vi "GageVolScale.vi"(2 "Voltage Scale":u16(ring)=4) -> (1 "Scaling Factor":dbl format="%.2f")   [LabVIEW 2022 SP3]
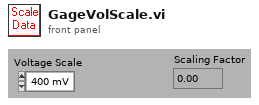
[diagram p1: front panel]
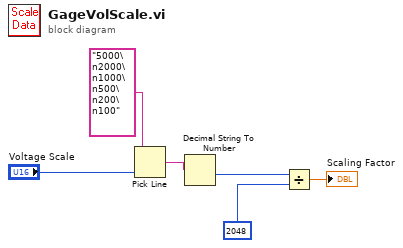
[diagram p0: block diagram]
diagram:
  n1 = Pick Line(multi-line string="5000\n2000\n1000\n500\n200\n100", line index="Voltage Scale") -> (output string=w5:string)  [unwired: 1 out]
  n2 = Decimal String To Number(string=w5) -> (number=w2:i32)  [unwired: 3 out]
  n3 = Divide(x=w2, y=2048) -> (x/y=→"Scaling Factor":dbl)
